vi "Knock Results Read.vi"(8 "error in":errorcluster, 9 "Device Outputs in":dbl[](array[numeric]), 10 "DCM Ref":refnum<class "DCM - RT.lvclass">, 11 "Knock in":T1={"Knock Enabled"=FALSE, "FIFO Indexes"={"Read"={"Knock"=[-1, -1, -1, -1, -1, -1, -1, -1, -1, -1, -1, -1, -1, -1, -1, -1], "Knock Intensity"=[-1, -1, -1, -1, -1, -1, -1, -1, -1, -1, -1, -1, -1, -1, -1, -1]}, "Write"={"Low Cutoff [Hz]"=5000, "High Cutoff [Hz]"=6000, "Threshold"=2, "Knock Start [CAD]"=0, "Knock End [CAD]"=0, "Reference Start [CAD]"=0, "Reference End [CAD]"=0}}, "Settings"={"Sensor Select"=[0, 0, 0, 0, 0, 0, 0, 0, 0, 0, 0, 0, 0, 0, 0, 0], "Cylinder Offset [CAD]"=[0.0, 0.0, 0.0, 0.0, 0.0, 0.0, 0.0, 0.0, 0.0, 0.0, 0.0, 0.0, 0.0, 0.0, 0.0, 0.0]}} {"Settings"."Sensor Select" items=["Sensor 1", "Sensor 2", "Sensor 3", "Sensor 4", "Sensor 5", "Sensor 6", "Sensor 7", "Sensor 8", "Sensor 9", "Sensor 10", "Sensor 11", "Sensor 12"]}) -> (0 "error out":errorcluster, 1 "Device Outputs out":dbl[](array[numeric]))   [LabVIEW 2016, in "DCM Engine.lvlib"]
uses:
  DCM Engine.lvlib
  Built/DCM Classes Packed/Pharlap/C/DCM-Classes.lvlibp/DCM/Rev0/RT/DCM - RT.lvclass
  Shared/Types/Knock.ctl
  Built/DCM Classes Packed/Pharlap/C/DCM-Classes.lvlibp/DCM/Tools/RT/DCM - RT - Tools.lvlib
  DCM Shared.lvlib
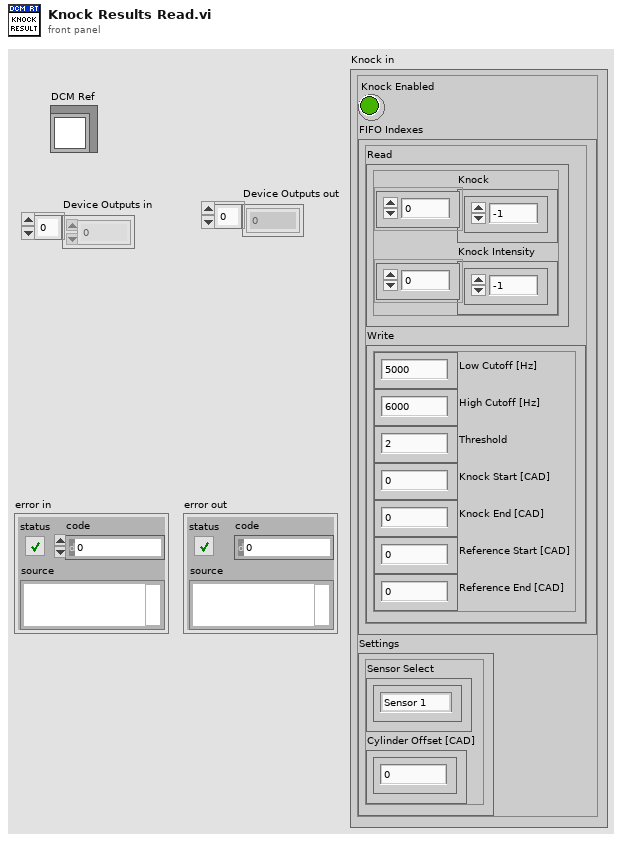
[diagram p1: front panel]
types:
  T1 = typedef "DCM Shared.lvlib/Knock.ctl" = cluster{"Knock Enabled":bool, "FIFO Indexes":cluster{"Read":cluster{"Knock":i32[], "Knock Intensity":i32[]}, "Write":cluster{"Low Cutoff [Hz]":i32, "High Cutoff [Hz]":i32, "Threshold":i32, "Knock Start [CAD]":i32, "Knock End [CAD]":i32, "Reference Start [CAD]":i32, "Reference End [CAD]":i32}}, "Settings":cluster{"Sensor Select":i32[], "Cylinder Offset [CAD]":sgl[]}}
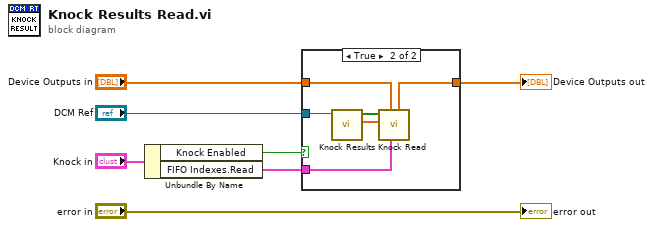
[diagram p0: block diagram]
diagram:
  n1 = Unbundle By Name("Knock in") -> ("Knock Enabled"=w1:bool, "FIFO Indexes.Read"=w2:cluster{"Knock":i32[], "Knock Intensity":i32[]})
  n2 = case shown="True" w1 {
    tunnel: "DCM Ref" -> [_ w14]
    tunnel: "Device Outputs in" -> [w8 w13]
    tunnel: [w8 w12] -> w4
    tunnel: w2 -> [_ w11]
    frame False {
    }
    frame True {
      n3 = call "Knock Results.vi"("DCM Reference"=w14) -> ("Knock Intensity"=w9:sgl[], "Knock"=w10:bool[])  [unwired: 9 in]
      n4 = call "Knock Read.vi"("FIFO Indexes.Read"=w11, "Device Outputs in"=w13, "Knock Intensity"=w9, "Knock"=w10) -> ("Device Outputs out"=w12:dbl[])  [unwired: 7 in]
    }
  }
  "Device Outputs out" <- w4
  "error out" <- "error in"
